vi "setUp.vi"(8 "error in (no error)":errorcluster, 11 "reference in":refnum<class "MyFirstTest.lvclass">) -> (0 "error out":errorcluster, 3 "reference in":refnum<class "MyFirstTest.lvclass">)   [LabVIEW 2013, in "MyFirstTest.lvclass"]
uses:
  MyFirstTest.lvclass
  MyFirstTest.lvclass/MyFirstTest.ctl
panel:
  # "Copyright © 2007 James Kring, Inc. All rights reserved.\n\nAuthor: Jim Kring [jim.kring@jameskring.com]\n\nThis library is provided \"AS IS\" ,WITHOUT WARRANTIES OR \nCONDITIONS OF ANY KIND, either express or implied.\n\nJames Kring, Inc. -- http://www.jameskring.com"
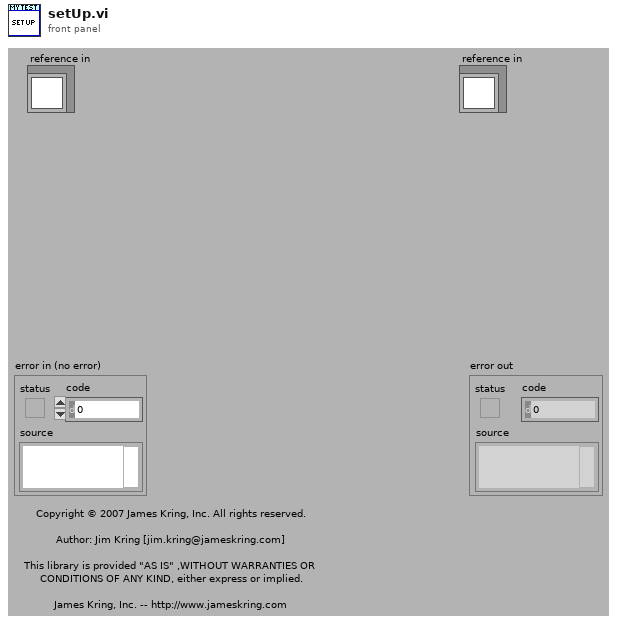
[diagram p1: front panel]
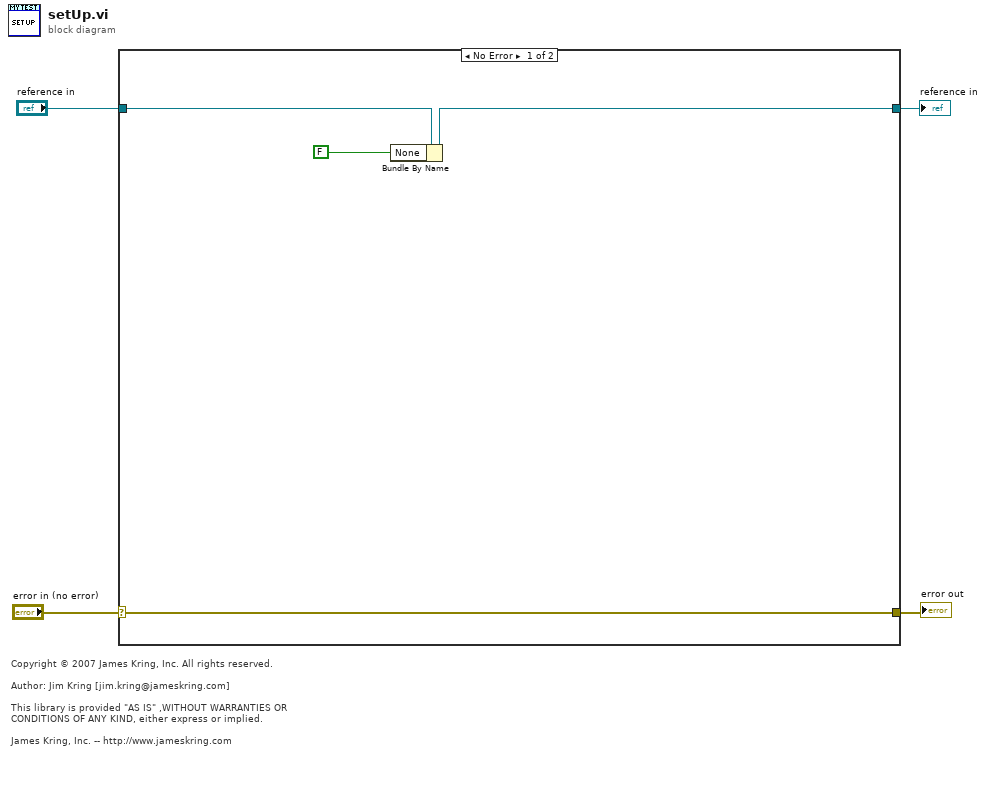
[diagram p0: block diagram]
diagram:
  # "Copyright © 2007 James Kring, Inc. All rights reserved.\n\nAuthor: Jim Kring [jim.kring@jameskring.com]\n\nThis library is provided \"AS IS\" ,WITHOUT WARRANTIES OR \nCONDITIONS OF ANY KIND, either express or implied.\n\nJames Kring, Inc. -- http://www.jameskring.com"
  n1 = case shown="No Error" "error in (no error)" {
    selector: "error in (no error)" -> [w5 w10]
    tunnel: [w5 w10] -> w3
    tunnel: [w6 w9] -> w1
    tunnel: "reference in" -> [w8 w9]
    frame No Error {
      n2 = Bundle By Name(cluster=w8, "None"=FALSE) -> (w6:refnum<class "MyFirstTest.lvclass">)
    }
    frame Error {
    }
  }
  "error out" <- w3
  "reference in" <- w1
